vi "Create From VI Reference.vi"(8 "error in (no error)":errorcluster, 10 "VI":refnum<vi>) -> (0 "error out":errorcluster, 3 "CSM-Helper.lvclass":refnum<class "CSM-Helper.lvclass">)   [LabVIEW 2020, in "CSM-Helper.lvclass"]
uses:
  CSM-Helper.lvclass
  CSM-Helper.lvclass/CSM-Helper.ctl
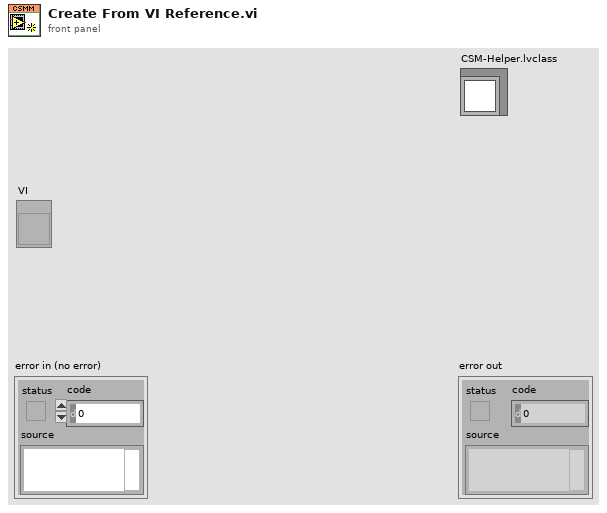
[diagram p1: front panel]
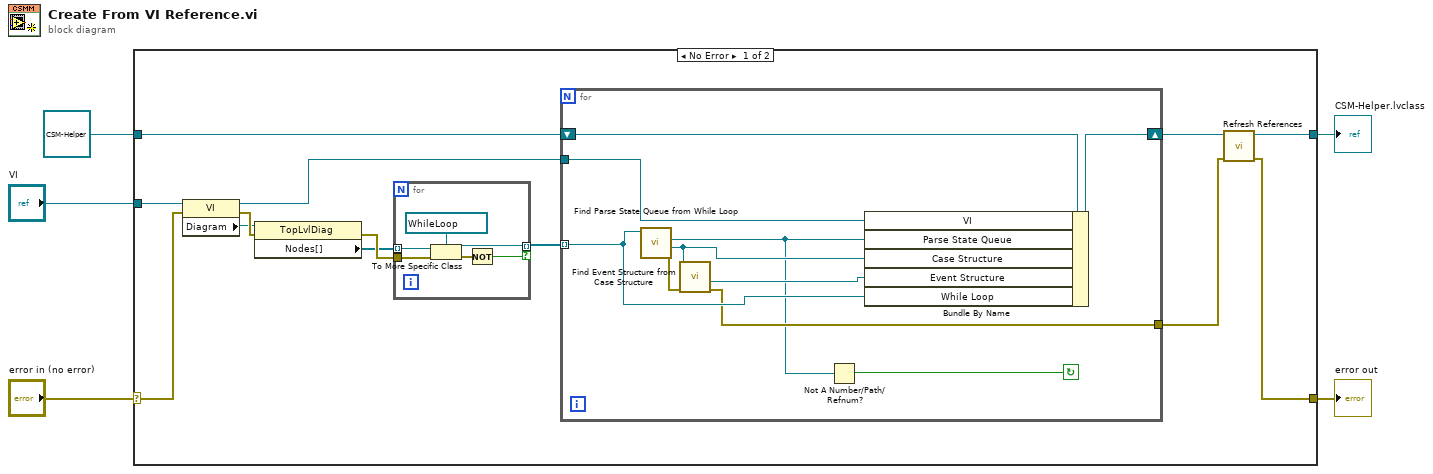
[diagram p0: block diagram]
diagram:
  n1 = case shown="No Error" "error in (no error)" {
    selector: "error in (no error)" -> [w13 w36]
    tunnel: [w9 w36] -> w4
    tunnel: [w10 w35] -> w2
    tunnel: refnum<class "CSM-Helper.lvclass"> refnum ("JKI SM") -> [w12 w35]
    tunnel: "VI" -> [w14 _]
    frame No Error {
      n2 = property class="VI"(reference=w14, error in=w13) -> (reference out=w7:refnum<vi>, error out=w18:errorcluster, "Diagram"=w15:refnum<vi>)
      n3 = property class="TopLvlDiag"(reference=w15, error in=w18) -> (error out=w17:errorcluster, "Nodes[]"=w16:refnum<vi>[])  [unwired: 1 out]
      n4 = for {
        tunnel: w16 -> [w33] mode=indexing
        tunnel: [w31] -> w8 mode=indexing if=w29
        tunnel: w17 -> [w32]
        n5 = To More Specific Class(target class=refnum<vi> refnum ("WLoop Refnum"), reference=w33, error in=w32) -> (specific class reference=w31:refnum<vi>, error out=w30:errorcluster)
        n6 = Not(x=w30) -> (.not. x?=w29:bool)
      }
      n7 = for {
        tunnel: w8 -> [w23] mode=indexing
        tunnel: w7 -> [w22]
        tunnel: [w21] -> w6
        shift-right: [w25] -> w11
        shift-left: w12 -> [w28]
        stop <- w19 continue-if-true
        n8 = call "Find Parse State Queue from While Loop.vi"("WhileLoop in"=w23) -> ("error out"=w27:errorcluster, "CaseStructure"=w26:refnum<vi>, "Parse State Queue"=w20:refnum<vi>)  [unwired: 7 in, 1 out]
        n9 = call "Find Event Structure from Case Structure.vi"("error in (no error)"=w27, "CaseStructure"=w26) -> ("error out"=w21:errorcluster, "EvntStruct Refnum"=w24:refnum<vi>)  [unwired: 8 in]
        n10 = Not A Number/Path/Refnum?(number/path/refnum=w20) -> (NaN/Path/Refnum?=w19:bool)
        n11 = Bundle By Name(cluster=w28, "VI"=w22, "Parse State Queue"=w20, "Case Structure"=w26, "Event Structure"=w24, "While Loop"=w23) -> (w25:refnum<class "CSM-Helper.lvclass">)
      }
      n12 = call "Refresh References.vi"("error in (no error)"=w6, "CSM-Helper in"=w11) -> ("error out"=w9:errorcluster, "CSM-Helper out"=w10:refnum<class "CSM-Helper.lvclass">)  [unwired: 8 in]
    }
    frame Error {
    }
  }
  "error out" <- w4
  "CSM-Helper.lvclass" <- w2
